vi "Car Wash.vi"() -> ()   [LabVIEW 2015]
uses:
  USB Template (LV 8.6)/Car Wash/Controls/Car Wash Indicators.ctl
  USB Template (LV 8.6)/Car Wash/Controls/Wash Options.ctl
  controls/state.ctl
  controls/Car wash data.ctl
  controls/times.ctl
  controls/timerstate.ctl
panel:
  out "error out":errorcluster
  in  "error in":errorcluster
  in  "Wash Options":T1
  in  "Start":bool
  out "Elapsed Time":dbl format="%0.2f"
  in  "stop":bool
  out "Wash Entry":bool
  in  "Car Position Slider":u8(slide) max=3 scale=0.0..4.0
  out "Car Wash Indicators":T2
  # "Entry Console"
  # "Car Wash Display"
  # "Car Position Simulation"
  # "Pre-Soak\nH-P Wash\nL-P Wax\nSpot Free Rinse"
  # "Underbody Wash\nBug Remover"
  # "Tire Shine\nAir Dry"
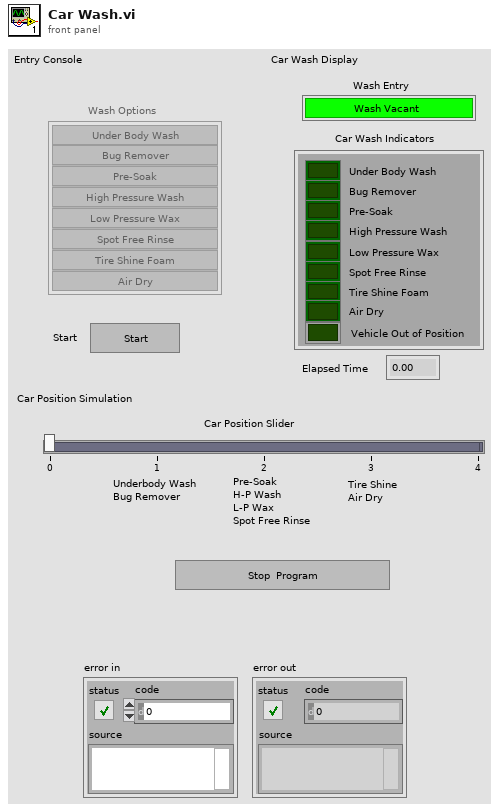
[diagram p1: front panel]
types:
  T1 = typedef "Wash Options.ctl" = cluster{"Underbody Wash":bool, "Bug Remover":bool, "Pre-Soak":bool, "High Pressure Wash":bool, "Low Pressure Wax":bool, "Spot Free Rinse":bool, "Tire Shine Foam":bool, "Air Dry":bool}
  T2 = typedef "Car Wash Indicators.ctl" = cluster{"Under Body Wash":bool, "Bug Remover":bool, "Pre-Soak":bool, "High Pressure Wash":bool, "Low Pressure Wax":bool, "Spot Free Rinse":bool, "Tire Shine Foam":bool, "Air Dry":bool, "Vehicle Out of Position":bool}
  T3 = typedef "state.ctl" = enum16{"End", "Reset", "Initialize", "Idle", "UBW", "TSF", "SFR", "LPW", "HPW", "P-S", "BR", "AD", "Error", "Exit"}
  T4 = enum8{"Enabled", "Disabled", "Disabled and Grayed Out"}
  T5 = typedef "timerstate.ctl" = enum16{"Stop", "Pause", "Start"}
  T6 = typedef "Car wash data.ctl" = cluster{"Wash Options":T1, "Car Wash Indicators":T2, "Wash Entry":bool, "Elapsed Time":dbl, "times":T7}
  T7 = typedef "times.ctl" = cluster{"UBW":dbl, "BR":dbl, "P-S":dbl, "HPW":dbl, "LPW":dbl, "SFR":dbl, "TSF":dbl, "AD":dbl}
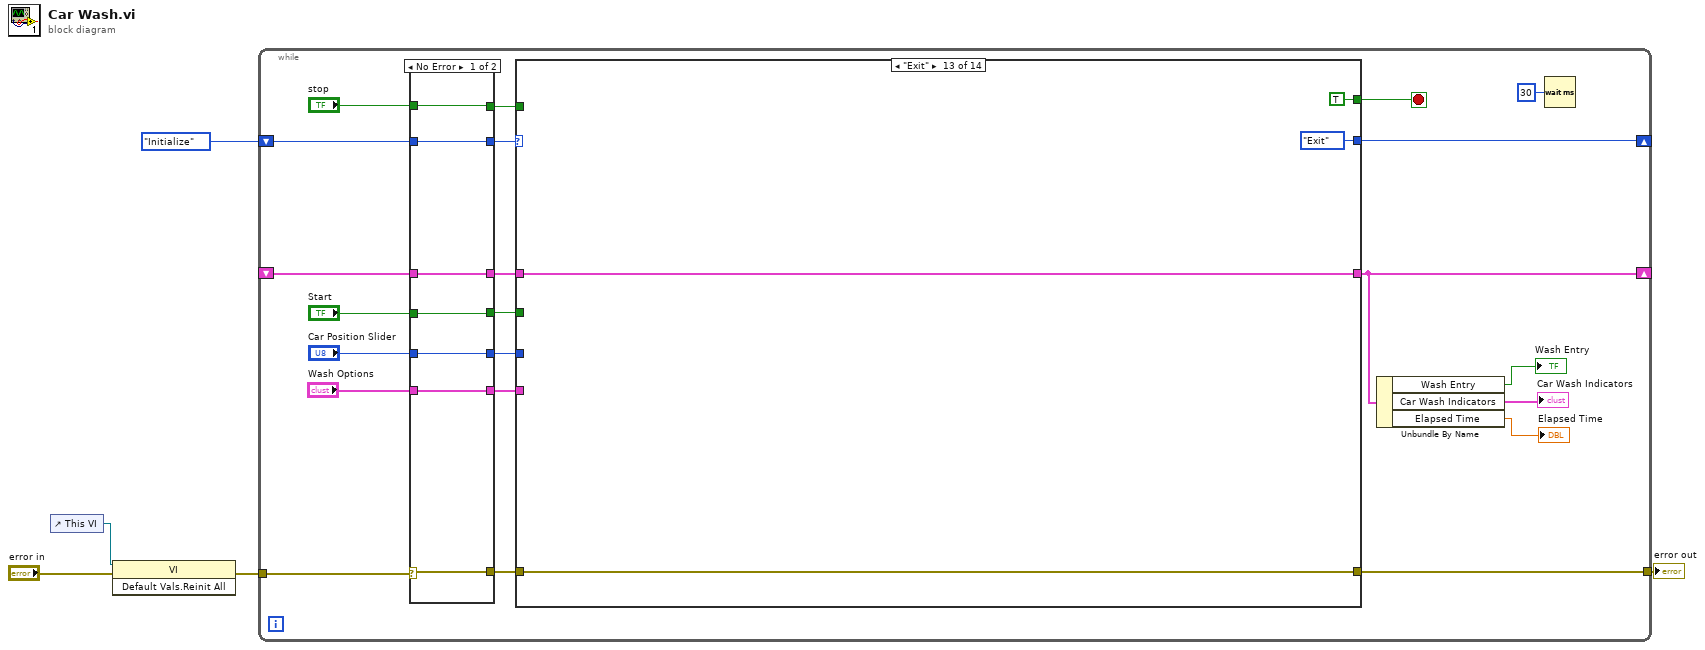
[diagram p0: block diagram]
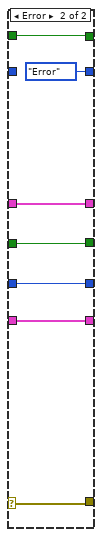
[diagram p2: hidden frame]
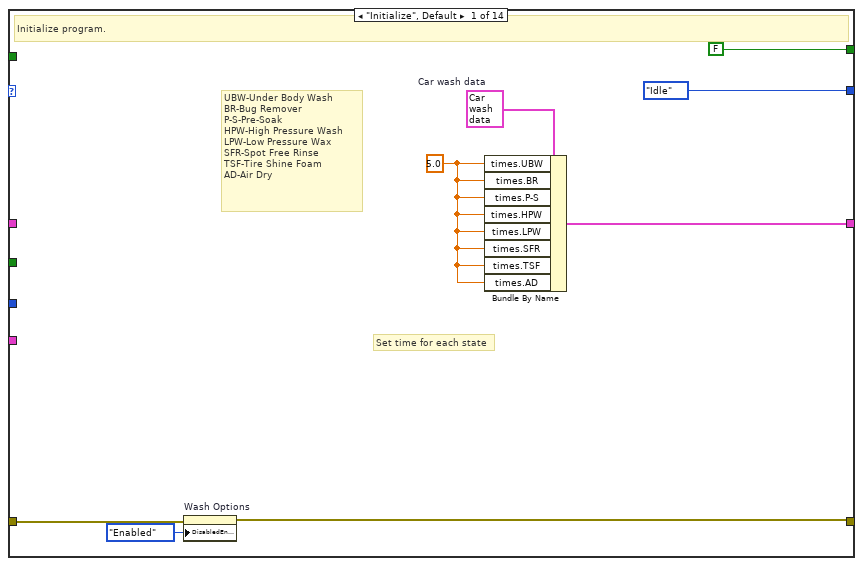
[diagram p3: hidden frame]
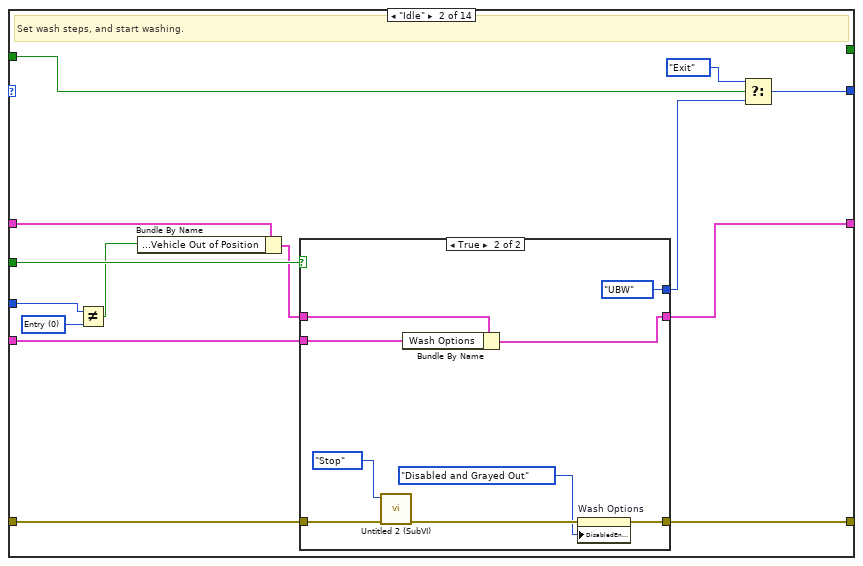
[diagram p4: hidden frame]
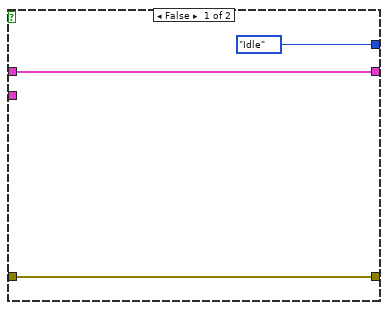
[diagram p5: hidden frame]
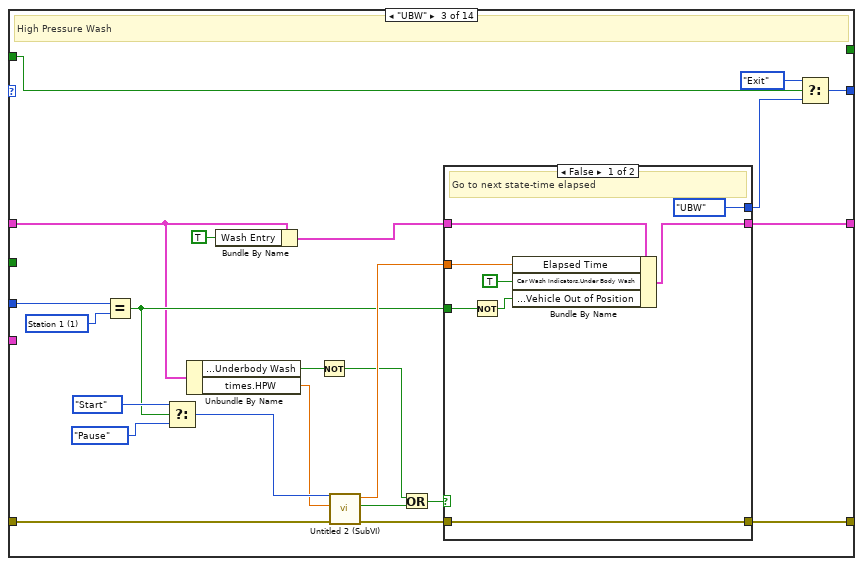
[diagram p6: hidden frame]
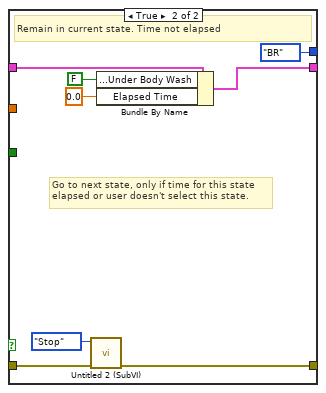
[diagram p7: hidden frame]
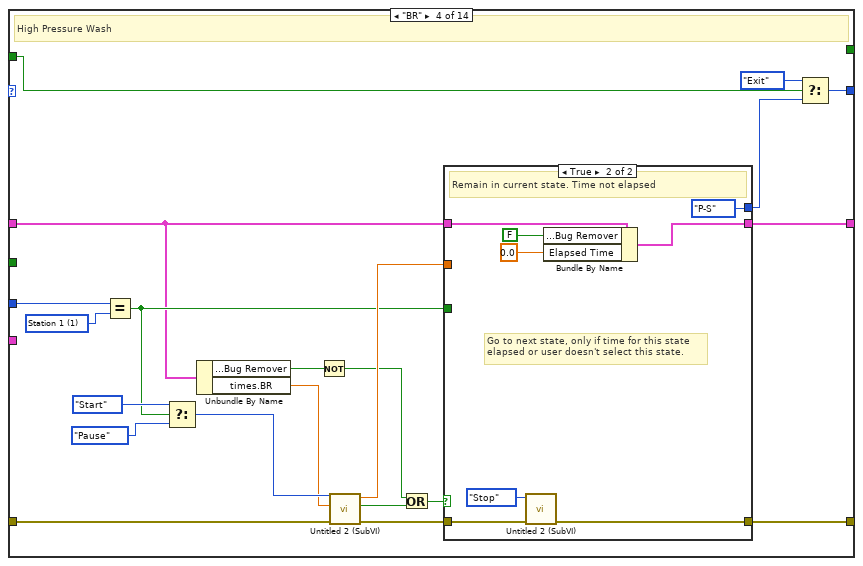
[diagram p8: hidden frame]
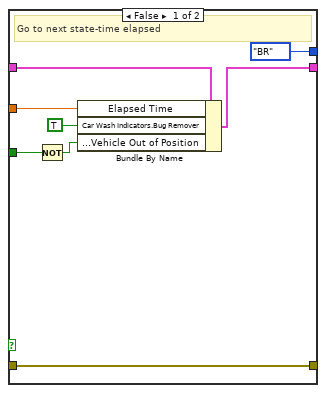
[diagram p9: hidden frame]
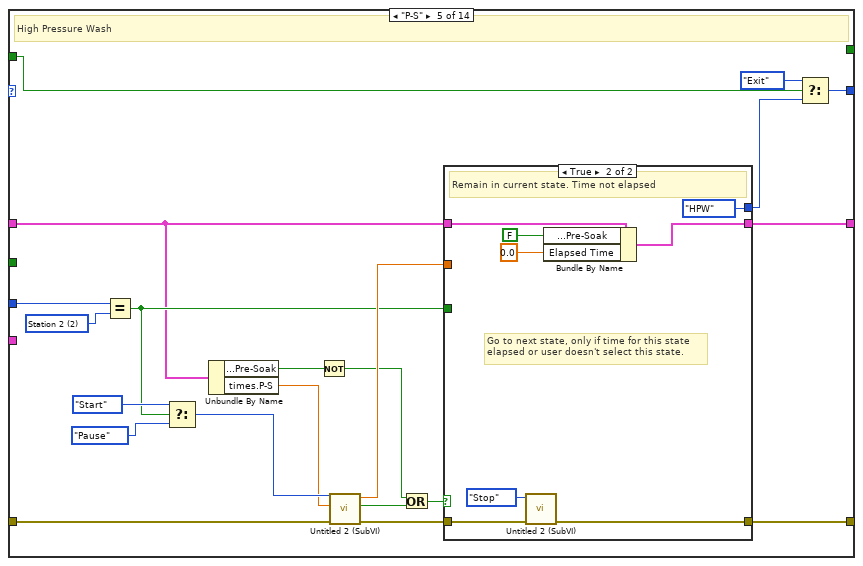
[diagram p10: hidden frame]
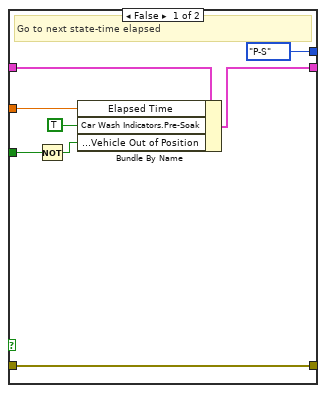
[diagram p11: hidden frame]
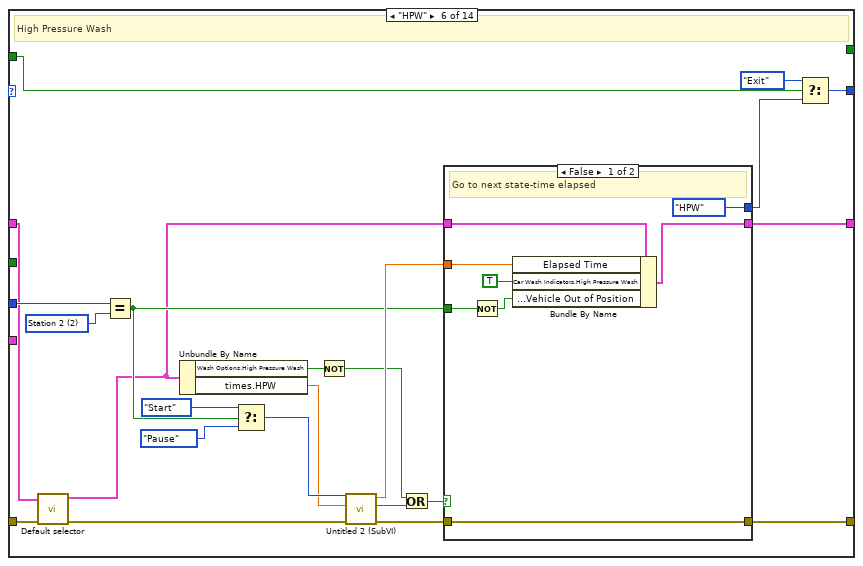
[diagram p12: hidden frame]
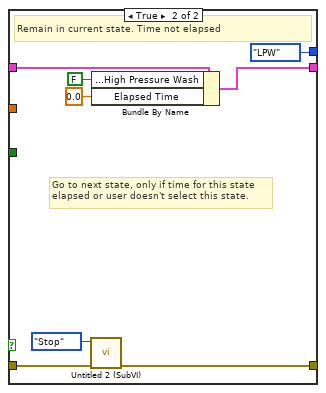
[diagram p13: hidden frame]
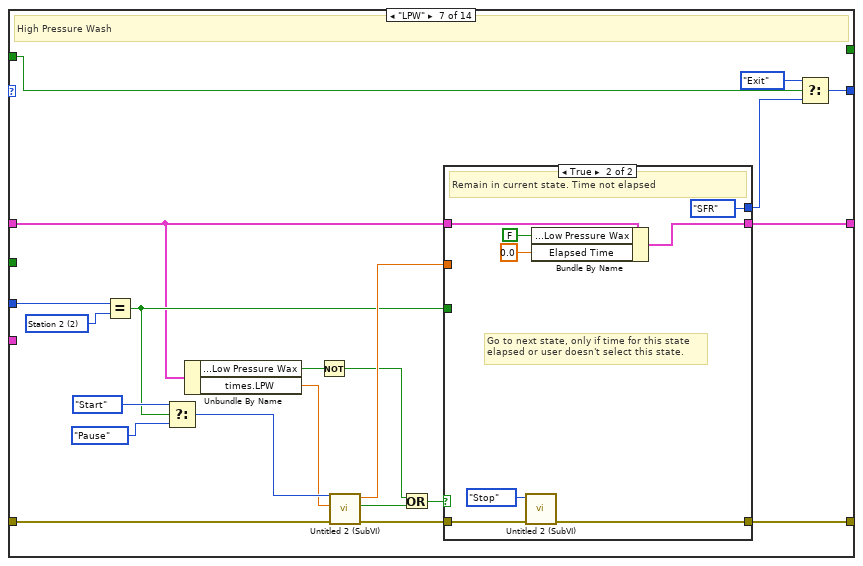
[diagram p14: hidden frame]
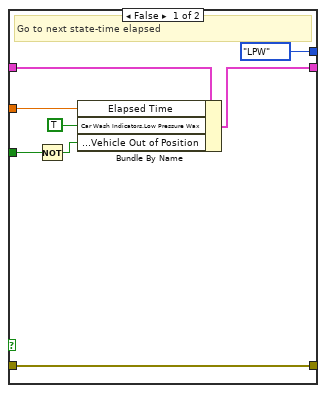
[diagram p15: hidden frame]
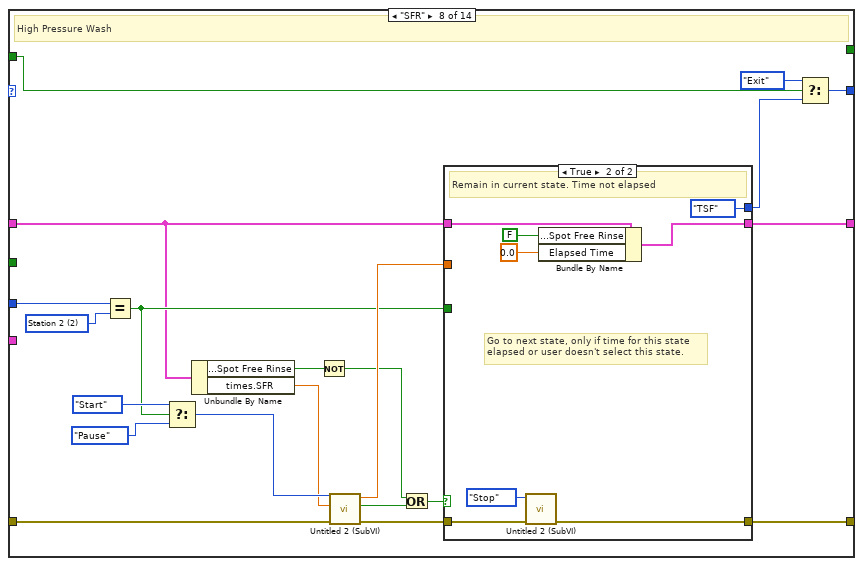
[diagram p16: hidden frame]
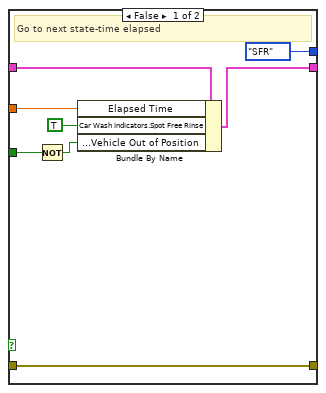
[diagram p17: hidden frame]
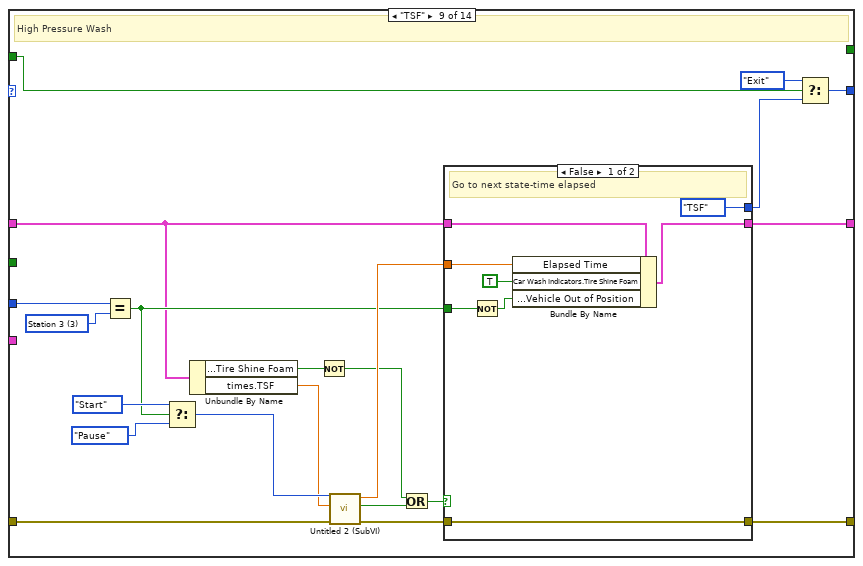
[diagram p18: hidden frame]
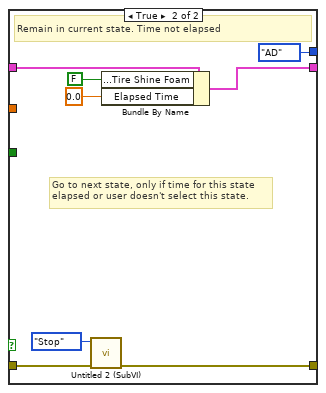
[diagram p19: hidden frame]
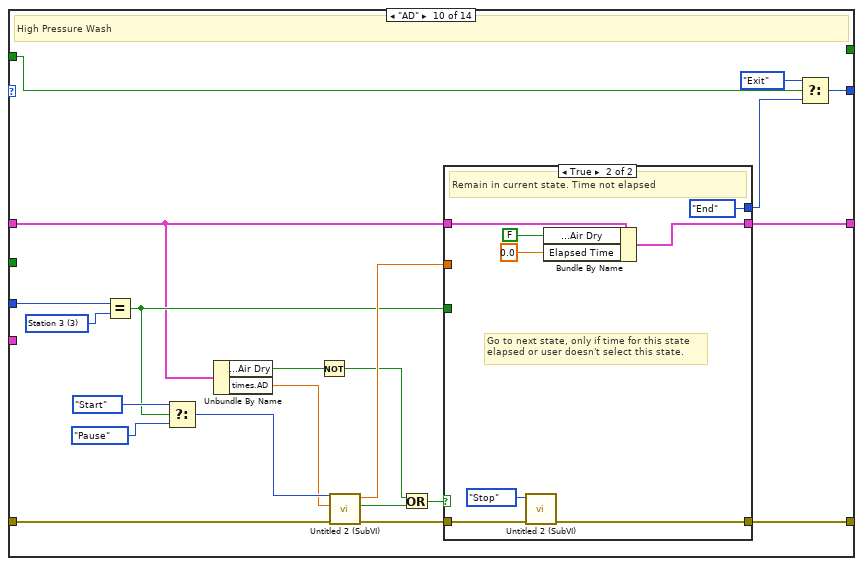
[diagram p20: hidden frame]
diagram:
  n1 = control-ref of="This VI"() -> (w3:refnum<vi>)
  n2 = invoke class="VI" method="Default Vals.Reinit All"(reference=w3, error in="error in") -> (error out=w2:errorcluster)  [unwired: 1 in, 2 out]
  n3 = while {
    shift-right: [w25] -> _
    shift-left: state."Initialize" ("state") -> [w19]
    tunnel: w2 -> [w23]
    tunnel: [w27] -> w4
    shift-right: [w10] -> _
    shift-left: _ -> [w22]
    stop <- w26 stop-if-true
    n4 = case shown="No Error" w23 {
      selector: w23 -> [w34 w40]
      tunnel: [w34 w40] -> w24
      tunnel: w22 -> [w33 w35]
      tunnel: [w33 w35] -> w21
      tunnel: [w32 state."Error" ("state")] -> w20
      tunnel: w19 -> [w32 _]
      tunnel: [w28 w39] -> w17
      tunnel: "stop" -> [w28 w39]
      tunnel: [w31 w38] -> w15
      tunnel: "Start" -> [w31 w38]
      tunnel: "Car Position Slider" -> [w30 w37]
      tunnel: [w30 w37] -> w13
      tunnel: "Wash Options" -> [w29 w36]
      tunnel: [w29 w36] -> w11
      frame No Error {
      }
      frame Error {
      }
    }
    n5 = case shown="\"Exit\"" w20 {
      tunnel: w24 -> [w44 w63 w96 w133 w170 w192 w246 w283 w320 w357 w377 w399 w405 w413]
      tunnel: [w43 w52 w84 w121 w158 w198 w234 w271 w308 w345 w376 w398 w405 w407] -> w27
      tunnel: [FALSE _ _ _ _ _ _ _ _ _ _ _ TRUE _] -> w26
      tunnel: [w47 w53 w89 w126 w163 w203 w239 w276 w313 w350 w382 w400 w404 w410] -> w10
      tunnel: [state."Idle" ("state") w54 w85 w122 w159 w199 w235 w272 w309 w346 w378 state."Exit" ("state") state."Exit" ("state") state."Idle" ("state")] -> w25
      tunnel: w21 -> [_ w60 w82 w115 w152 w191 w228 w265 w302 w339 w384 w400 w404 w410]
      tunnel: w17 -> [_ w57 w88 w125 w162 w202 w238 w275 w312 w349 w381 _ _ _]
      tunnel: w15 -> [_ w59 _ _ _ _ _ _ _ _ _ _ _ _]
      tunnel: w13 -> [_ w61 w98 w135 w172 w211 w248 w285 w322 w359 w385 _ _ _]
      tunnel: w11 -> [_ w50 _ _ _ _ _ _ _ _ _ _ _ _]
      frame "Initialize", Default {
        w46 = 5.0 ("times.UBW")
        w49 = T6 {"Wash Options"={"Underbody Wash"=FALSE, "Bug Remover"=FALSE, "Pre-Soak"=FALSE, "High Pressure Wash"=FALSE, "Low Pressure Wax"=FALSE, "Spot Free Rinse"=FALSE, "Tire Shine Foam"=FALSE, "Air Dry"=FALSE}, "Car Wash Indicators"={"Under Body Wash"=FALSE, "Bug Remover"=FALSE, "Pre-Soak"=FALSE, "High Pressure Wash"=FALSE, "Low Pressure Wax"=FALSE, "Spot Free Rinse"=FALSE, "Tire Shine Foam"=FALSE, "Air Dry"=FALSE, "Vehicle Out of Position"=FALSE}, "Wash Entry"=FALSE, "Elapsed Time"=0.0, "times"={"UBW"=0.0, "BR"=0.0, "P-S"=0.0, "HPW"=0.0, "LPW"=0.0, "SFR"=0.0, "TSF"=0.0, "AD"=0.0}}  # Car wash data
        # "UBW-Under Body Wash\nBR-Bug Remover\nP-S-Pre-Soak\nHPW-High Pressure Wash\nLPW-Low Pressure Wax\nSFR-Spot Free Rinse\nTSF-Tire Shine Foam\nAD-Air Dry"
        # "Set time for each state"
        # "Initialize program."
        n6 = property on="Wash Options" class="Clust (strict)"(error in=w44, "DisabledEnum"=T4."Enabled" ("Disabled")) -> (error out=w43:errorcluster)  [unwired: 1 in, 1 out]
        n7 = Bundle By Name(cluster=w49, "times.UBW"=w46, "times.BR"=w46, "times.P-S"=w46, "times.HPW"=w46, "times.LPW"=w46, "times.SFR"=w46, "times.TSF"=w46, "times.AD"=w46) -> (w47:T6)
      }
      frame "Idle" {
        w62 = u8 0 items=["Entry", "Station 1", "Station 2", "Station 3", "Exit"] ("Car Position Slider")
        # "Set wash steps, and start washing."
        n8 = Not Equal?(x=w61, y=w62) -> (x != y?=w51:bool)
        n9 = Bundle By Name(cluster=w60, "Car Wash Indicators.Vehicle Out of Position"=w51) -> (w58:T6)
        n10 = case shown="True" w59 {
          tunnel: w63 -> [w64 w75]
          tunnel: w58 -> [w65 w73]
          tunnel: [state."Idle" ("state") state."UBW" ("state")] -> w56
          tunnel: [w65 w71] -> w53
          tunnel: [w64 w68] -> w52
          tunnel: w50 -> [_ w72]
          frame False {
          }
          frame True {
            n11 = call "Untitled 2 (SubVI).vi"("error in"=w75, "timerstate"=timerstate."Stop") -> ("error out"=w69:errorcluster)  [unwired: 7 in, 2 out]
            n12 = Bundle By Name(cluster=w73, "Wash Options"=w72) -> (w71:T6)
            n13 = property on="Wash Options" class="Clust (strict)"(error in=w69, "DisabledEnum"=T4."Disabled and Grayed Out" ("Disabled")) -> (error out=w68:errorcluster)  [unwired: 1 in, 1 out]
          }
        }
        n14 = Select(t=state."Exit", s=w57, f=w56) -> (s? t:f=w54:T3)
      }
      frame "UBW" {
        w97 = u8 1 items=["Entry", "Station 1", "Station 2", "Station 3", "Exit"] ("Car Position Slider")
        # "High Pressure Wash"
        n15 = Equal?(x=w98, y=w97) -> (x = y?=w83:bool)
        n16 = Select(t=timerstate."Start" ("timerstate"), s=w83, f=timerstate."Pause" ("timerstate")) -> (s? t:f=w93:T5)
        n17 = Unbundle By Name(w82) -> ("Wash Options.Underbody Wash"=w77:bool, "times.HPW"=w92:dbl)
        n18 = Bundle By Name(cluster=w82, "Wash Entry"=TRUE) -> (w81:T6)
        n19 = Not(x=w77) -> (.not. x?=w76:bool)
        n20 = call "Untitled 2 (SubVI).vi"("error in"=w96, "limit"=w92, "timerstate"=w93) -> ("error out"=w91:errorcluster, "limit reached"=w78:bool, "elapsed"=w90:dbl)  [unwired: 6 in]
        n21 = Or(x=w76, y=w78) -> (x .or. y?=w79:bool)
        n22 = case shown="False" w79 {
          tunnel: w91 -> [w101 w114]
          tunnel: w81 -> [w106 w111]
          tunnel: w90 -> [w105 _]
          tunnel: [w103 w108] -> w89
          tunnel: [state."UBW" ("state") state."BR" ("state")] -> w87
          tunnel: [w101 w113] -> w84
          tunnel: w83 -> [w100 _]
          frame False {
            # "Go to next state-time elapsed"
            n23 = Not(x=w100) -> (.not. x?=w99:bool)
            n24 = Bundle By Name(cluster=w106, "Elapsed Time"=w105, "Car Wash Indicators.Under Body Wash"=TRUE ("Car Wash Indicators.High Pressure Wash"), "Car Wash Indicators.Vehicle Out of Position"=w99) -> (w103:T6)
          }
          frame True {
            # "Go to next state, only if time for this state \nelapsed or user doesn't select this state."
            # "Remain in current state. Time not elapsed"
            n25 = call "Untitled 2 (SubVI).vi"("error in"=w114, "timerstate"=timerstate."Stop") -> ("error out"=w113:errorcluster)  [unwired: 7 in, 2 out]
            n26 = Bundle By Name(cluster=w111, "Car Wash Indicators.Under Body Wash"=FALSE ("Wash Options.High Pressure Wash"), "Elapsed Time"=0.0) -> (w108:T6)
          }
        }
        n27 = Select(t=state."Exit", s=w88, f=w87) -> (s? t:f=w85:T3)
      }
      frame "BR" {
        w134 = u8 1 items=["Entry", "Station 1", "Station 2", "Station 3", "Exit"] ("Car Position Slider")
        # "High Pressure Wash"
        n28 = Equal?(x=w135, y=w134) -> (x = y?=w120:bool)
        n29 = Select(t=timerstate."Start" ("timerstate"), s=w120, f=timerstate."Pause" ("timerstate")) -> (s? t:f=w130:T5)
        n30 = Unbundle By Name(w115) -> ("Wash Options.Bug Remover"=w117:bool, "times.BR"=w129:dbl)
        n31 = Not(x=w117) -> (.not. x?=w116:bool)
        n32 = call "Untitled 2 (SubVI).vi"("error in"=w133, "limit"=w129, "timerstate"=w130) -> ("error out"=w128:errorcluster, "limit reached"=w118:bool, "elapsed"=w127:dbl)  [unwired: 6 in]
        n33 = Or(x=w116, y=w118) -> (x .or. y?=w119:bool)
        n34 = case shown="True" w119 {
          tunnel: w128 -> [w138 w151]
          tunnel: w115 -> [w143 w148]
          tunnel: w127 -> [w142 _]
          tunnel: [w140 w145] -> w126
          tunnel: [state."BR" ("state") state."P-S" ("state")] -> w124
          tunnel: [w138 w150] -> w121
          tunnel: w120 -> [w137 _]
          frame False {
            # "Go to next state-time elapsed"
            n35 = Not(x=w137) -> (.not. x?=w136:bool)
            n36 = Bundle By Name(cluster=w143, "Elapsed Time"=w142, "Car Wash Indicators.Bug Remover"=TRUE ("Car Wash Indicators.High Pressure Wash"), "Car Wash Indicators.Vehicle Out of Position"=w136) -> (w140:T6)
          }
          frame True {
            # "Go to next state, only if time for this state \nelapsed or user doesn't select this state."
            # "Remain in current state. Time not elapsed"
            n37 = call "Untitled 2 (SubVI).vi"("error in"=w151, "timerstate"=timerstate."Stop") -> ("error out"=w150:errorcluster)  [unwired: 7 in, 2 out]
            n38 = Bundle By Name(cluster=w148, "Car Wash Indicators.Bug Remover"=FALSE ("Wash Options.High Pressure Wash"), "Elapsed Time"=0.0) -> (w145:T6)
          }
        }
        n39 = Select(t=state."Exit", s=w125, f=w124) -> (s? t:f=w122:T3)
      }
      frame "P-S" {
        w171 = u8 2 items=["Entry", "Station 1", "Station 2", "Station 3", "Exit"] ("Car Position Slider")
        # "High Pressure Wash"
        n40 = Equal?(x=w172, y=w171) -> (x = y?=w157:bool)
        n41 = Select(t=timerstate."Start" ("timerstate"), s=w157, f=timerstate."Pause" ("timerstate")) -> (s? t:f=w167:T5)
        n42 = Unbundle By Name(w152) -> ("Wash Options.Pre-Soak"=w154:bool, "times.P-S"=w166:dbl)
        n43 = Not(x=w154) -> (.not. x?=w153:bool)
        n44 = call "Untitled 2 (SubVI).vi"("error in"=w170, "limit"=w166, "timerstate"=w167) -> ("error out"=w165:errorcluster, "limit reached"=w155:bool, "elapsed"=w164:dbl)  [unwired: 6 in]
        n45 = Or(x=w153, y=w155) -> (x .or. y?=w156:bool)
        n46 = case shown="True" w156 {
          tunnel: w165 -> [w175 w188]
          tunnel: w152 -> [w180 w185]
          tunnel: w164 -> [w179 _]
          tunnel: [w177 w182] -> w163
          tunnel: [state."P-S" ("state") state."HPW" ("state")] -> w161
          tunnel: [w175 w187] -> w158
          tunnel: w157 -> [w174 _]
          frame False {
            # "Go to next state-time elapsed"
            n47 = Not(x=w174) -> (.not. x?=w173:bool)
            n48 = Bundle By Name(cluster=w180, "Elapsed Time"=w179, "Car Wash Indicators.Pre-Soak"=TRUE ("Car Wash Indicators.High Pressure Wash"), "Car Wash Indicators.Vehicle Out of Position"=w173) -> (w177:T6)
          }
          frame True {
            # "Go to next state, only if time for this state \nelapsed or user doesn't select this state."
            # "Remain in current state. Time not elapsed"
            n49 = call "Untitled 2 (SubVI).vi"("error in"=w188, "timerstate"=timerstate."Stop") -> ("error out"=w187:errorcluster)  [unwired: 7 in, 2 out]
            n50 = Bundle By Name(cluster=w185, "Car Wash Indicators.Pre-Soak"=FALSE ("Wash Options.High Pressure Wash"), "Elapsed Time"=0.0) -> (w182:T6)
          }
        }
        n51 = Select(t=state."Exit", s=w162, f=w161) -> (s? t:f=w159:T3)
      }
      frame "HPW" {
        w210 = u8 2 items=["Entry", "Station 1", "Station 2", "Station 3", "Exit"] ("Car Position Slider")
        # "High Pressure Wash"
        n52 = call "Default selector.vi"("error in"=w192, "Car wash data"=w191) -> ("error out"=w189:errorcluster, "output cluster"=w190:T6)  [unwired: 8 in]
        n53 = Equal?(x=w211, y=w210) -> (x = y?=w197:bool)
        n54 = Unbundle By Name(w190) -> ("Wash Options.High Pressure Wash"=w194:bool, "times.HPW"=w206:dbl)
        n55 = Select(t=timerstate."Start" ("timerstate"), s=w197, f=timerstate."Pause" ("timerstate")) -> (s? t:f=w207:T5)
        n56 = Not(x=w194) -> (.not. x?=w193:bool)
        n57 = call "Untitled 2 (SubVI).vi"("error in"=w189, "limit"=w206, "timerstate"=w207) -> ("error out"=w205:errorcluster, "limit reached"=w195:bool, "elapsed"=w204:dbl)  [unwired: 6 in]
        n58 = Or(x=w193, y=w195) -> (x .or. y?=w196:bool)
        n59 = case shown="False" w196 {
          tunnel: w205 -> [w214 w227]
          tunnel: w190 -> [w219 w224]
          tunnel: w204 -> [w218 _]
          tunnel: [w216 w221] -> w203
          tunnel: [state."HPW" ("state") state."LPW" ("state")] -> w201
          tunnel: [w214 w226] -> w198
          tunnel: w197 -> [w213 _]
          frame False {
            # "Go to next state-time elapsed"
            n60 = Not(x=w213) -> (.not. x?=w212:bool)
            n61 = Bundle By Name(cluster=w219, "Elapsed Time"=w218, "Car Wash Indicators.High Pressure Wash"=TRUE, "Car Wash Indicators.Vehicle Out of Position"=w212) -> (w216:T6)
          }
          frame True {
            # "Go to next state, only if time for this state \nelapsed or user doesn't select this state."
            # "Remain in current state. Time not elapsed"
            n62 = call "Untitled 2 (SubVI).vi"("error in"=w227, "timerstate"=timerstate."Stop") -> ("error out"=w226:errorcluster)  [unwired: 7 in, 2 out]
            n63 = Bundle By Name(cluster=w224, "Car Wash Indicators.High Pressure Wash"=FALSE ("Wash Options.High Pressure Wash"), "Elapsed Time"=0.0) -> (w221:T6)
          }
        }
        n64 = Select(t=state."Exit", s=w202, f=w201) -> (s? t:f=w199:T3)
      }
      frame "LPW" {
        w247 = u8 2 items=["Entry", "Station 1", "Station 2", "Station 3", "Exit"] ("Car Position Slider")
        # "High Pressure Wash"
        n65 = Equal?(x=w248, y=w247) -> (x = y?=w233:bool)
        n66 = Select(t=timerstate."Start" ("timerstate"), s=w233, f=timerstate."Pause" ("timerstate")) -> (s? t:f=w243:T5)
        n67 = Unbundle By Name(w228) -> ("Wash Options.Low Pressure Wax"=w230:bool, "times.LPW"=w242:dbl)
        n68 = Not(x=w230) -> (.not. x?=w229:bool)
        n69 = call "Untitled 2 (SubVI).vi"("error in"=w246, "limit"=w242, "timerstate"=w243) -> ("error out"=w241:errorcluster, "limit reached"=w231:bool, "elapsed"=w240:dbl)  [unwired: 6 in]
        n70 = Or(x=w229, y=w231) -> (x .or. y?=w232:bool)
        n71 = case shown="True" w232 {
          tunnel: w241 -> [w251 w264]
          tunnel: w228 -> [w256 w261]
          tunnel: w240 -> [w255 _]
          tunnel: [w253 w258] -> w239
          tunnel: [state."LPW" ("state") state."SFR" ("state")] -> w237
          tunnel: [w251 w263] -> w234
          tunnel: w233 -> [w250 _]
          frame False {
            # "Go to next state-time elapsed"
            n72 = Not(x=w250) -> (.not. x?=w249:bool)
            n73 = Bundle By Name(cluster=w256, "Elapsed Time"=w255, "Car Wash Indicators.Low Pressure Wax"=TRUE ("Car Wash Indicators.High Pressure Wash"), "Car Wash Indicators.Vehicle Out of Position"=w249) -> (w253:T6)
          }
          frame True {
            # "Go to next state, only if time for this state \nelapsed or user doesn't select this state."
            # "Remain in current state. Time not elapsed"
            n74 = call "Untitled 2 (SubVI).vi"("error in"=w264, "timerstate"=timerstate."Stop") -> ("error out"=w263:errorcluster)  [unwired: 7 in, 2 out]
            n75 = Bundle By Name(cluster=w261, "Car Wash Indicators.Low Pressure Wax"=FALSE ("Wash Options.High Pressure Wash"), "Elapsed Time"=0.0) -> (w258:T6)
          }
        }
        n76 = Select(t=state."Exit", s=w238, f=w237) -> (s? t:f=w235:T3)
      }
      frame "SFR" {
        w284 = u8 2 items=["Entry", "Station 1", "Station 2", "Station 3", "Exit"] ("Car Position Slider")
        # "High Pressure Wash"
        n77 = Equal?(x=w285, y=w284) -> (x = y?=w270:bool)
        n78 = Select(t=timerstate."Start" ("timerstate"), s=w270, f=timerstate."Pause" ("timerstate")) -> (s? t:f=w280:T5)
        n79 = Unbundle By Name(w265) -> ("Wash Options.Spot Free Rinse"=w267:bool, "times.SFR"=w279:dbl)
        n80 = Not(x=w267) -> (.not. x?=w266:bool)
        n81 = call "Untitled 2 (SubVI).vi"("error in"=w283, "limit"=w279, "timerstate"=w280) -> ("error out"=w278:errorcluster, "limit reached"=w268:bool, "elapsed"=w277:dbl)  [unwired: 6 in]
        n82 = Or(x=w266, y=w268) -> (x .or. y?=w269:bool)
        n83 = case shown="True" w269 {
          tunnel: w278 -> [w288 w301]
          tunnel: w265 -> [w293 w298]
          tunnel: w277 -> [w292 _]
          tunnel: [w290 w295] -> w276
          tunnel: [state."SFR" ("state") state."TSF" ("state")] -> w274
          tunnel: [w288 w300] -> w271
          tunnel: w270 -> [w287 _]
          frame False {
            # "Go to next state-time elapsed"
            n84 = Not(x=w287) -> (.not. x?=w286:bool)
            n85 = Bundle By Name(cluster=w293, "Elapsed Time"=w292, "Car Wash Indicators.Spot Free Rinse"=TRUE ("Car Wash Indicators.High Pressure Wash"), "Car Wash Indicators.Vehicle Out of Position"=w286) -> (w290:T6)
          }
          frame True {
            # "Go to next state, only if time for this state \nelapsed or user doesn't select this state."
            # "Remain in current state. Time not elapsed"
            n86 = call "Untitled 2 (SubVI).vi"("error in"=w301, "timerstate"=timerstate."Stop") -> ("error out"=w300:errorcluster)  [unwired: 7 in, 2 out]
            n87 = Bundle By Name(cluster=w298, "Car Wash Indicators.Spot Free Rinse"=FALSE ("Wash Options.High Pressure Wash"), "Elapsed Time"=0.0) -> (w295:T6)
          }
        }
        n88 = Select(t=state."Exit", s=w275, f=w274) -> (s? t:f=w272:T3)
      }
      frame "TSF" {
        w321 = u8 3 items=["Entry", "Station 1", "Station 2", "Station 3", "Exit"] ("Car Position Slider")
        # "High Pressure Wash"
        n89 = Equal?(x=w322, y=w321) -> (x = y?=w307:bool)
        n90 = Select(t=timerstate."Start" ("timerstate"), s=w307, f=timerstate."Pause" ("timerstate")) -> (s? t:f=w317:T5)
        n91 = Unbundle By Name(w302) -> ("Wash Options.Tire Shine Foam"=w304:bool, "times.TSF"=w316:dbl)
        n92 = Not(x=w304) -> (.not. x?=w303:bool)
        n93 = call "Untitled 2 (SubVI).vi"("error in"=w320, "limit"=w316, "timerstate"=w317) -> ("error out"=w315:errorcluster, "limit reached"=w305:bool, "elapsed"=w314:dbl)  [unwired: 6 in]
        n94 = Or(x=w303, y=w305) -> (x .or. y?=w306:bool)
        n95 = case shown="False" w306 {
          tunnel: w315 -> [w325 w338]
          tunnel: w302 -> [w330 w335]
          tunnel: w314 -> [w329 _]
          tunnel: [w327 w332] -> w313
          tunnel: [state."TSF" ("state") state."AD" ("state")] -> w311
          tunnel: [w325 w337] -> w308
          tunnel: w307 -> [w324 _]
          frame False {
            # "Go to next state-time elapsed"
            n96 = Not(x=w324) -> (.not. x?=w323:bool)
            n97 = Bundle By Name(cluster=w330, "Elapsed Time"=w329, "Car Wash Indicators.Tire Shine Foam"=TRUE ("Car Wash Indicators.High Pressure Wash"), "Car Wash Indicators.Vehicle Out of Position"=w323) -> (w327:T6)
          }
          frame True {
            # "Go to next state, only if time for this state \nelapsed or user doesn't select this state."
            # "Remain in current state. Time not elapsed"
            n98 = call "Untitled 2 (SubVI).vi"("error in"=w338, "timerstate"=timerstate."Stop") -> ("error out"=w337:errorcluster)  [unwired: 7 in, 2 out]
            n99 = Bundle By Name(cluster=w335, "Car Wash Indicators.Tire Shine Foam"=FALSE ("Wash Options.High Pressure Wash"), "Elapsed Time"=0.0) -> (w332:T6)
          }
        }
        n100 = Select(t=state."Exit", s=w312, f=w311) -> (s? t:f=w309:T3)
      }
      frame "AD" {
        w358 = u8 3 items=["Entry", "Station 1", "Station 2", "Station 3", "Exit"] ("Car Position Slider")
        # "High Pressure Wash"
        n101 = Equal?(x=w359, y=w358) -> (x = y?=w344:bool)
        n102 = Select(t=timerstate."Start" ("timerstate"), s=w344, f=timerstate."Pause" ("timerstate")) -> (s? t:f=w354:T5)
        n103 = Unbundle By Name(w339) -> ("Wash Options.Air Dry"=w341:bool, "times.AD"=w353:dbl)
        n104 = Not(x=w341) -> (.not. x?=w340:bool)
        n105 = call "Untitled 2 (SubVI).vi"("error in"=w357, "limit"=w353, "timerstate"=w354) -> ("error out"=w352:errorcluster, "limit reached"=w342:bool, "elapsed"=w351:dbl)  [unwired: 6 in]
        n106 = Or(x=w340, y=w342) -> (x .or. y?=w343:bool)
        n107 = case shown="True" w343 {
          tunnel: w352 -> [w362 w375]
          tunnel: w339 -> [w367 w372]
          tunnel: w351 -> [w366 _]
          tunnel: [w364 w369] -> w350
          tunnel: [state."AD" ("state") state."End" ("state")] -> w348
          tunnel: [w362 w374] -> w345
          tunnel: w344 -> [w361 _]
          frame False {
            # "Go to next state-time elapsed"
            n108 = Not(x=w361) -> (.not. x?=w360:bool)
            n109 = Bundle By Name(cluster=w367, "Elapsed Time"=w366, "Car Wash Indicators.Air Dry"=TRUE ("Car Wash Indicators.High Pressure Wash"), "Car Wash Indicators.Vehicle Out of Position"=w360) -> (w364:T6)
          }
          frame True {
            # "Go to next state, only if time for this state \nelapsed or user doesn't select this state."
            # "Remain in current state. Time not elapsed"
            n110 = call "Untitled 2 (SubVI).vi"("error in"=w375, "timerstate"=timerstate."Stop") -> ("error out"=w374:errorcluster)  [unwired: 7 in, 2 out]
            n111 = Bundle By Name(cluster=w372, "Car Wash Indicators.Air Dry"=FALSE ("Wash Options.High Pressure Wash"), "Elapsed Time"=0.0) -> (w369:T6)
          }
        }
        n112 = Select(t=state."Exit", s=w349, f=w348) -> (s? t:f=w346:T3)
      }
      frame "End" {
        w386 = u8 4 items=["Entry", "Station 1", "Station 2", "Station 3", "Exit"] ("Car Position Slider")
        n113 = Equal?(x=w385, y=w386) -> (x = y?=w383:bool)
        n114 = case shown="True" w383 {
          tunnel: w384 -> [w391 w396]
          tunnel: [w389 w395] -> w382
          tunnel: [state."End" ("state") state."Reset" ("state")] -> w379
          tunnel: w377 -> [w387 w393]
          tunnel: [w387 w393] -> w376
          frame False {
            n115 = Bundle By Name(cluster=w391, "Car Wash Indicators.Vehicle Out of Position"=TRUE) -> (w389:T6)
          }
          frame True {
            w394 = FALSE ("Car Wash Indicators.Vehicle Out of Position")
            n116 = Bundle By Name(cluster=w396, "Car Wash Indicators.Vehicle Out of Position"=w394, "Wash Entry"=w394) -> (w395:T6)
            n117 = Wait (ms)(milliseconds to wait=u32 50) -> ()  [unwired: 1 out]
          }
        }
        n118 = Select(t=state."Exit" ("state"), s=w381, f=w379) -> (s? t:f=w378:T3)
      }
      frame "Error" {
        n119 = call <vilib>:"Simple Error Handler.vi"("error in (no error)"=w399) -> ("error out"=w398:errorcluster)  [unwired: 4 in, 4 out]
      }
      frame "Exit" {
      }
      frame "Reset" {
        w406 = u8 0 items=["Entry", "Station 1", "Station 2", "Station 3", "Exit"] ("Car Position Slider")
        n120 = control-ref of="This VI"() -> (w414:refnum<vi>)
        n121 = invoke class="VI" method="Default Vals.Reinit All"(reference=w414, error in=w413) -> (error out=w412:errorcluster)  [unwired: 1 in, 2 out]
        n122 = property on="Wash Options" class="Clust (strict)"(error in=w412, "DisabledEnum"=T4."Enabled" ("Disabled")) -> (error out=w408:errorcluster)  [unwired: 1 in, 1 out]
        n123 = property on="Car Position Slider" class="Slide (strict)"(error in=w408, "Val(Sgnl)"=w406) -> (error out=w407:errorcluster)  [unwired: 1 in, 1 out]
      }
    }
    n124 = Unbundle By Name(w10) -> ("Wash Entry"=→"Wash Entry":bool, "Car Wash Indicators"=→"Car Wash Indicators":T2, "Elapsed Time"=→"Elapsed Time":dbl)
    n125 = Wait (ms)(milliseconds to wait=u32 30) -> ()  [unwired: 1 out]
  }
  "error out" <- w4
